vi "Close.vi"(8 "error in (no error)":errorcluster, 10 "Msg in":T1, 11 "FakePressureController in":refnum<class "MagAnalysis_Online.lvclass">) -> (0 "error out":errorcluster, 1 "new command":string, 2 "Msg out":T1, 3 "FakePressureController out":refnum<class "MagAnalysis_Online.lvclass">)   [LabVIEW 2020, in "MagAnalysis_Online.lvclass"]
uses:
  MagAnalysis_Online.lvclass
  DriverMsg.ctl
  specClustercommandTypdef.ctl
  MagAnalysis_Online.lvclass/MagAnalysis_Online.ctl
  source/Device Drivers/BaseDriver/BaseDriver.lvclass
  NI_Vision_Acquisition_Software.lvlib
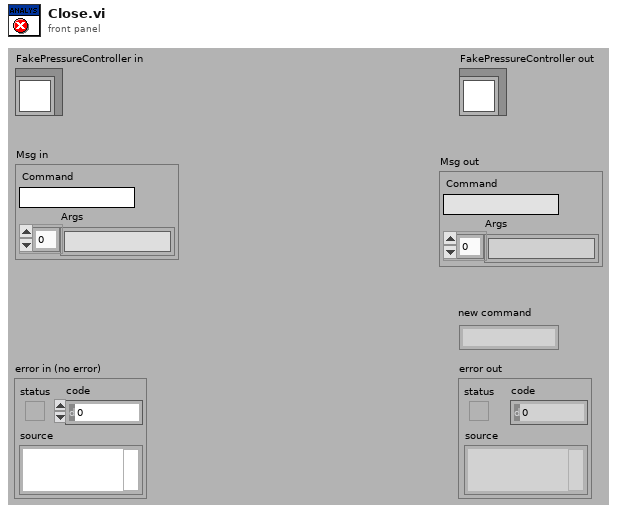
[diagram p1: front panel]
types:
  T1 = typedef "DriverMsg.ctl" = cluster{"Command":string, "Args":string[]}
  T2 = typedef "specClustercommandTypdef.ctl" = enum16{"init", "addCluster", "read", "clear"}
  T3 = typedef "IMAQ Image.ctl" = refnum<image>
  T4 = typedef "MagAnalysis_Online.lvclass/analysis_data_typdef.ctl" = cluster{"cam0":T3, "cam1":T3, "cam2":T3, "cam3":T3}
  T5 = typedef "bgImages_tyudef.ctl" = cluster{"cam 0":T3, "cam 1":T3, "cam 2":T3, "cam 3":T3}
  T6 = typedef "IMAQdx.ctl" = refnum<k21>
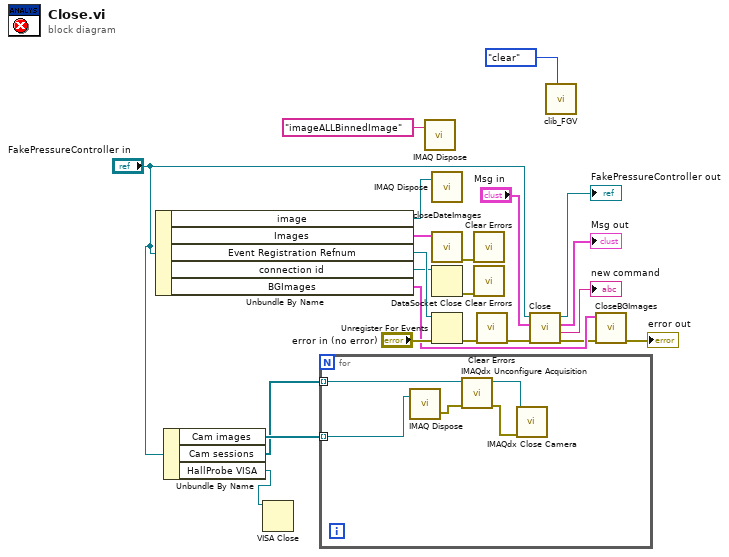
[diagram p0: block diagram]
diagram:
  n1 = Unbundle By Name("FakePressureController in") -> ("image"=w9:T3, "Images"=w6:T4, "Event Registration Refnum"=w18:refnum<event-registration>, "connection id"=w14:refnum<k13>, "BGImages"=w12:T5)
  n2 = Unbundle By Name("FakePressureController in") -> ("Cam images"=w3:T3[], "Cam sessions"=w2:T6[], "HallProbe VISA"=w1:refnum<visa-resource-name>)
  n3 = VISA Close(VISA resource name=w1) -> ()  [unwired: 1 in, 1 out]
  n4 = for {
    tunnel: w3 -> [w24] mode=indexing
    tunnel: w2 -> [w23] mode=indexing
    n5 = call "IMAQ Dispose"("Image"=w24) -> ("error out"=w25:errorcluster)  [unwired: 5 in]
    n6 = call "IMAQdx Unconfigure Acquisition.vi"("error in"=w25, "Session In"=w23) -> ("error out"=w27:errorcluster, "Session Out"=w26:T6)  [unwired: 8 in]
    n7 = call "IMAQdx Close Camera.vi"("error in"=w27, "Session In"=w26) -> ()  [unwired: 9 in, 1 out]
  }
  n8 = call "IMAQ Dispose"("Image"="imageALLBinnedImage" ("Image Name")) -> ()  [unwired: 5 in, 1 out]
  n9 = call "IMAQ Dispose"("Image"=w9) -> ()  [unwired: 5 in, 1 out]
  n10 = call "closeDateImages.vi"("data"=w6) -> ("error out"=w7:errorcluster)  [unwired: 10 in]
  n11 = DataSocket Close(11:w14) -> (0:w13:errorcluster)  [unwired: 2 in, 1 out]
  n12 = Unregister For Events(event registration refnum=w18, error in="error in (no error)") -> (error out=w15:errorcluster)
  n13 = call "Clear Errors.vi"("error in (no error)"=w7) -> ()  [unwired: 5 in, 2 out]
  n14 = call "Clear Errors.vi"("error in (no error)"=w13) -> ()  [unwired: 5 in, 2 out]
  n15 = call "Clear Errors.vi"("error in (no error)"=w15) -> ("error out"=w16:errorcluster)  [unwired: 5 in, 1 out]
  n16 = call-parent "Close.vi"("error in (no error)"=w16, "Msg in"="Msg in", "BaseDriver in"="FakePressureController in") -> ("error out"=w11:errorcluster, "new command"=→"new command":string, "Msg out"=→"Msg out":T1, "BaseDriver out"=→"FakePressureController out":refnum<class "MagAnalysis_Online.lvclass">)  [unwired: 5 in]
  n17 = call "clib_FGV.vi"("command"=specClustercommandTypdef."clear") -> ()  [unwired: 9 in, 2 out]
  n18 = call "CloseBGImages.vi"("error in (no error)"=w11, "BGImages"=w12) -> ("error out"=→"error out":errorcluster)  [unwired: 9 in]
